vi "Teleop-Sub-CameraControl.vi"(11 "Axes":dbl[](array[numeric])) -> ()   [LabVIEW 2016]
doc: "This VI accepts Joystick Axes data and uses that to point the camera using the camera Servo."
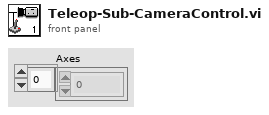
[diagram p1: front panel]
types:
  T1 = typedef "WPI_ServoDeviceRef.ctl" = cluster{"DeviceStatus":errorcluster, "PWM Channel":T2, "DeadBand":T3}
  T2 = typedef "FPGA_DIOPWMChannel.ctl" = enum8{"PWM 0", "PWM 1", "PWM 2", "PWM 3", "PWM 4", "PWM 5", "PWM 6", "PWM 7", "PWM 8", "PWM 9", "PWM MXP 0", "PWM MXP 1", "PWM MXP 2", "PWM MXP 3", "PWM MXP 4", "PWM MXP 5", "PWM MXP 6", "PWM MXP 7", "PWM MXP 8", "PWM MXP 9", "Invalid"}
  T3 = typedef "WPI_PWMDeadband.ctl" = cluster{"Name":string, "maxPositivePwm":i32, "minPositivePwm":i32, "centerPwm":i32, "maxNegativePwm":i32, "minNegativePwm":i32, "angularRange":u16}
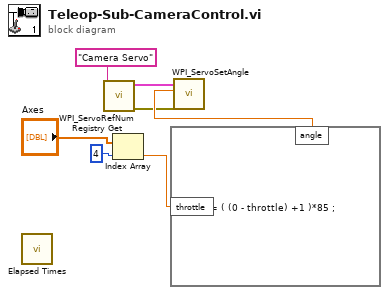
[diagram p0: block diagram]
diagram:
  n1 = call "Elapsed Times.vi"() -> ()  [unwired: 3 in, 1 out]
  n2 = call <vilib>:"WPI_ServoRefNum Registry Get.vi"("refnum name"="Camera Servo") -> ("error out"=w3:errorcluster, "ServoDeviceRef"=w4:T1)  [unwired: 9 in]
  n3 = Index Array(array="Axes", index=4) -> (element=w6:dbl)
  n4 = formula code="angle = ( (0 - throttle) +1 )*85 ;"("throttle"=w6) -> ("angle"=w7:dbl)
  n5 = call <vilib>:"WPI_ServoSetAngle.vi"("error in (no error)"=w3, "Angle"=w7, "ServoDeviceRef"=w4) -> ()  [unwired: 7 in, 2 out]
